vi "Save Libraries and Projects.vi"(8 "error in (no error)":errorcluster) -> (0 "error out":errorcluster)   [LabVIEW 2021, in "Converter.lvlib"]
uses:
  Converter.lvlib
  Converter Reusables/Converter Reusables.lvlib
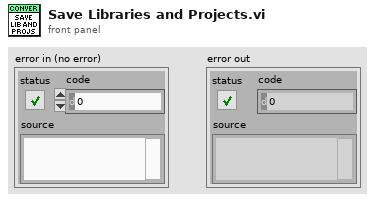
[diagram p1: front panel]
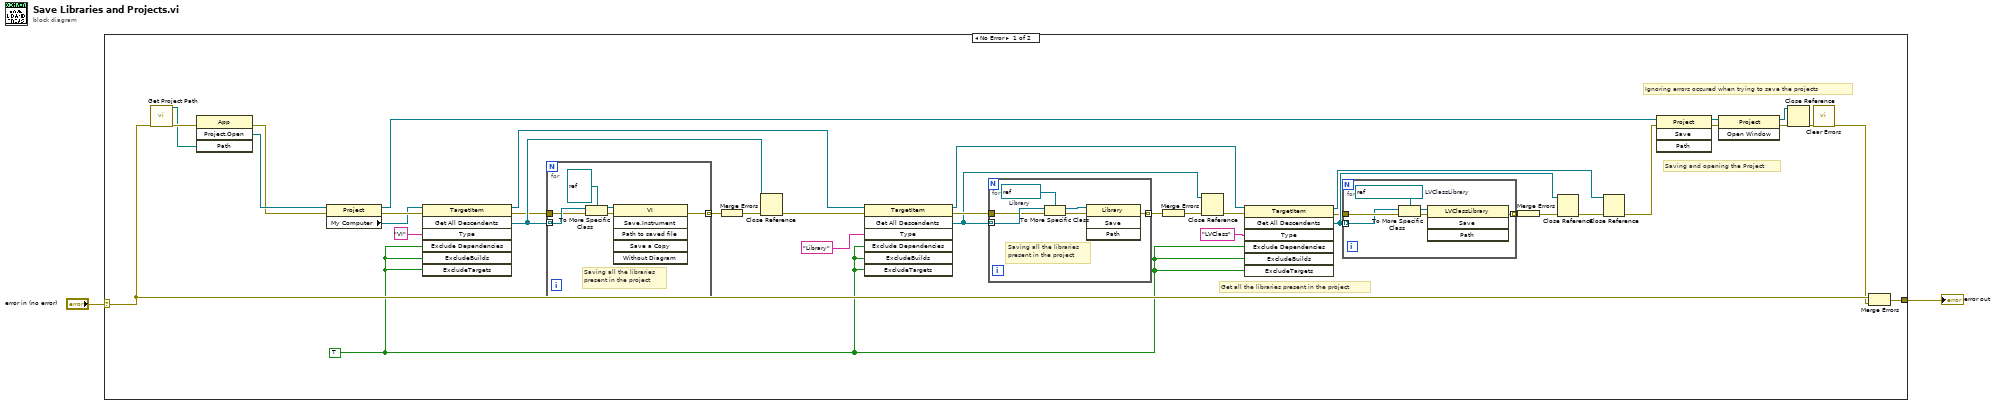
[diagram p0: block diagram]
diagram:
  n1 = case shown="No Error" "error in (no error)" {
    selector: "error in (no error)" -> [w27 w59]
    tunnel: [w28 w59] -> w2
    frame No Error {
      w4 = TRUE ("ExcludeDependencies")
      # "Get all the libraries present in the project"
      # "Saving and opening the Project"
      # "Ignoring errors occured when trying to save the projects"
      n2 = call "Get Project Path.vi"("error in (no error)"=w27) -> ("Project Path Out"=w35:path, "error out"=w36:errorcluster)  [unwired: 13 in]
      n3 = invoke class="App" method="Project.Open"(error in=w36, "Path"=w35) -> (error out=w30:errorcluster, "Project:Open"=w32:refnum<vi>)  [unwired: 2 in, 2 out]
      n4 = property class="Project"(reference=w32, error in=w30) -> (reference out=w26:refnum<vi>, error out=w8:errorcluster, "My Computer"=w6:refnum<vi>)
      n5 = invoke class="TargetItem" method="Get All Descendents"(reference=w6, error in=w8, "Type"="VI", "Exclude Dependencies"=w4, "ExcludeBuilds"=w4, "ExcludeTargets"=w4) -> (reference out=w5:refnum<vi>, error out=w9:errorcluster, "All Descendents"=w13:refnum<vi>[])  [unwired: 1 in, 4 out]
      n6 = for {
        tunnel: w13 -> [w46] mode=indexing
        tunnel: w9 -> [w43]
        tunnel: [w44] -> w11 mode=indexing
        # "Saving all the libraries \npresent in the project"
        n7 = To More Specific Class(target class=refnum<vi> refnum ("vi reference"), reference=w46, error in=w43) -> (specific class reference=w45:refnum<vi>, error out=w42:errorcluster)
        n8 = invoke class="VI" method="Save.Instrument"(reference=w45, error in=w42) -> (error out=w44:errorcluster)  [unwired: 4 in, 5 out]
      }
      n9 = Merge Errors(w11) -> (w12:errorcluster)
      n10 = Close Reference(reference=w13, error in (no error)=w12) -> (error out=w7:errorcluster)
      n11 = invoke class="TargetItem" method="Get All Descendents"(reference=w5, error in=w7, "Type"="Library", "Exclude Dependencies"=w4, "ExcludeBuilds"=w4, "ExcludeTargets"=w4) -> (reference out=w17:refnum<vi>, error out=w34:errorcluster, "All Descendents"=w24:refnum<vi>[])  [unwired: 1 in, 4 out]
      n12 = for {
        tunnel: w24 -> [w58] mode=indexing
        tunnel: w34 -> [w54]
        tunnel: [w55] -> w31 mode=indexing
        w57 = refnum<vi> refnum  # Library
        # "Saving all the libraries \npresent in the project"
        n13 = To More Specific Class(target class=w57, reference=w58, error in=w54) -> (specific class reference=w56:refnum<vi>, error out=w53:errorcluster)
        n14 = invoke class="Library" method="Save"(reference=w56, error in=w53) -> (error out=w55:errorcluster)  [unwired: 2 in, 3 out]
      }
      n15 = Merge Errors(w31) -> (w25:errorcluster)
      n16 = Close Reference(reference=w24, error in (no error)=w25) -> (error out=w18:errorcluster)
      n17 = invoke class="TargetItem" method="Get All Descendents"(reference=w17, error in=w18, "Type"="LVClass", "Exclude Dependencies"=w4, "ExcludeBuilds"=w4, "ExcludeTargets"=w4) -> (reference out=w16:refnum<vi>, error out=w19:errorcluster, "All Descendents"=w23:refnum<vi>[])  [unwired: 1 in, 4 out]
      n18 = for {
        tunnel: w23 -> [w47] mode=indexing
        tunnel: w19 -> [w49]
        tunnel: [w50] -> w21 mode=indexing
        w52 = refnum<vi> refnum  # LVClassLibrary
        n19 = To More Specific Class(target class=w52, reference=w47, error in=w49) -> (specific class reference=w51:refnum<vi>, error out=w48:errorcluster)
        n20 = invoke class="LVClassLibrary" method="Save"(reference=w51, error in=w48) -> (error out=w50:errorcluster)  [unwired: 2 in, 3 out]
      }
      n21 = Merge Errors(w21) -> (w22:errorcluster)
      n22 = Close Reference(reference=w23, error in (no error)=w22) -> (error out=w15:errorcluster)
      n23 = Close Reference(reference=w16, error in (no error)=w15) -> (error out=w14:errorcluster)
      n24 = invoke class="Project" method="Save"(reference=w26, error in=w14) -> (reference out=w37:refnum<vi>, error out=w39:errorcluster)  [unwired: 2 in, 2 out]
      n25 = invoke class="Project" method="Open Window"(reference=w37, error in=w39) -> (reference out=w38:refnum<vi>, error out=w40:errorcluster)  [unwired: 1 in, 1 out]
      n26 = Close Reference(reference=w38, error in (no error)=w40) -> (error out=w29:errorcluster)
      n27 = call <vilib>:"Clear Errors.vi"("error in (no error)"=w29) -> ("error out"=w3:errorcluster)  [unwired: 5 in, 1 out]
      n28 = Merge Errors(w27, w3) -> (w28:errorcluster)
    }
    frame Error {
    }
  }
  "error out" <- w2
